vi "Refocus.vi"(8 "Error In":errorcluster, 11 "Focus and Tracking":T1) -> (0 "Error Out":errorcluster, 2 "Error":bool)   [LabVIEW 2012, in "Targeting Unit.lvlib"]
uses:
  Targeting Unit.lvlib
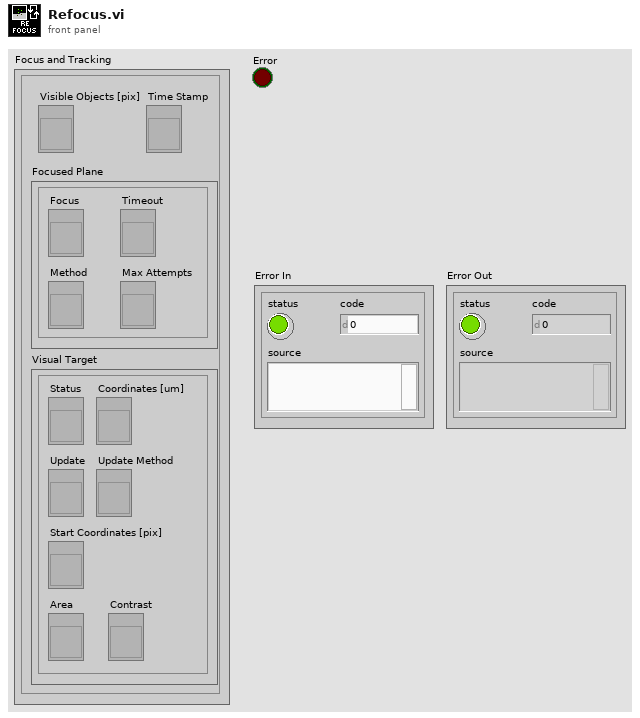
[diagram p1: front panel]
types:
  T1 = cluster{"Focused Plane":cluster{"Focus":refnum<vi>, "Timeout":refnum<vi>, "Max Attempts":refnum<vi>, "Method":refnum<vi>}, "Time Stamp":refnum<vi>, "Visual Target":cluster{"Coordinates [um]":refnum<vi>, "Status":refnum<vi>, "Update":refnum<vi>, "Update Method":refnum<vi>, "Start Coordinates [pix]":refnum<vi>, "Area":refnum<vi>, "Contrast":refnum<vi>}, "Visible Objects [pix]":refnum<vi>}
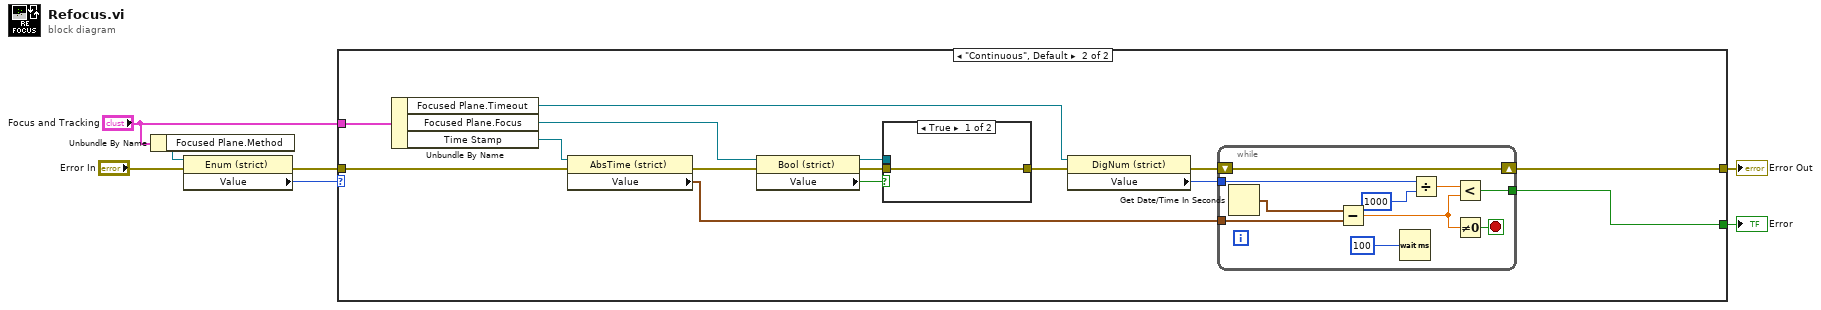
[diagram p0: block diagram]
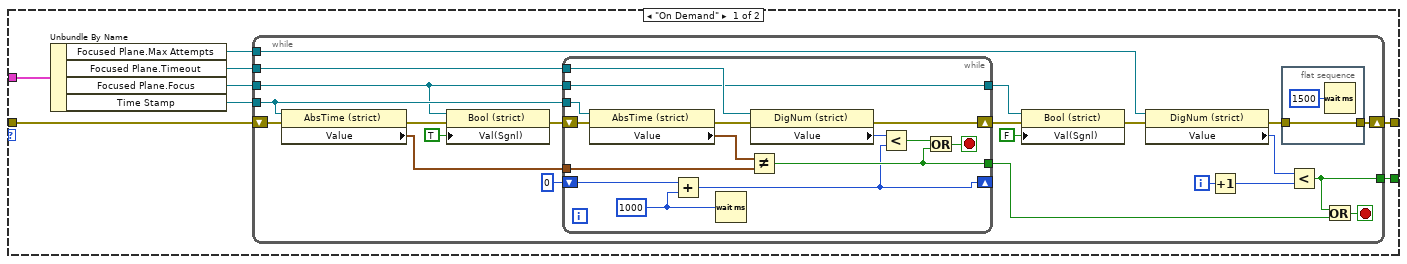
[diagram p2: hidden frame]
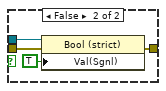
[diagram p3: hidden frame]
diagram:
  n1 = Unbundle By Name("Focus and Tracking") -> ("Focused Plane.Method"=w5:refnum<vi>)
  n2 = property class="Enum (strict)"(reference=w5, error in="Error In") -> (error out=w3:errorcluster, "Value"=w2:enum16{"Continuous", "On Demand"})  [unwired: 1 out]
  n3 = case shown="\"Continuous\", Default" w2 {
    tunnel: [w15 w69] -> w7
    tunnel: w3 -> [w14 w66]
    tunnel: [w13 w68] -> w6
    tunnel: "Focus and Tracking" -> [w12 w67]
    frame "On Demand" {
      n4 = Unbundle By Name(w12) -> ("Focused Plane.Max Attempts"=w8:refnum<vi>, "Focused Plane.Timeout"=w9:refnum<vi>, "Focused Plane.Focus"=w10:refnum<vi>, "Time Stamp"=w11:refnum<vi>)
      n5 = while {
        tunnel: w10 -> [w19]
        tunnel: w11 -> [w20]
        shift-right: [w17] -> w13
        shift-left: w14 -> [w23]
        tunnel: w8 -> [w29]
        tunnel: w9 -> [w27]
        tunnel: [w24] -> w15
        i -> [w32]
        stop <- w30 stop-if-true
        n6 = property class="AbsTime (strict)"(reference=w20, error in=w23) -> (error out=w22:errorcluster, "Value"=w21:timestamp)  [unwired: 1 out]
        n7 = property class="Bool (strict)"(reference=w19, error in=w22, "Val(Sgnl)"=TRUE ("Value (Signaling)")) -> (error out=w36:errorcluster)  [unwired: 1 out]
        n8 = while {
          tunnel: w21 -> [w53]
          tunnel: w20 -> [w52]
          shift-right: [w42] -> _
          shift-left: u32 0 -> [w43]
          tunnel: [w50] -> w18
          shift-right: [w48] -> w34
          shift-left: w36 -> [w54]
          tunnel: w27 -> [w47]
          tunnel: [w46] -> w26
          tunnel: w19 -> [w46]
          stop <- w51 stop-if-true
          w40 = u32 1000 ("milliseconds to wait")
          n9 = property class="AbsTime (strict)"(reference=w52, error in=w54) -> (error out=w49:errorcluster, "Value"=w41:timestamp)  [unwired: 1 out]
          n10 = Add(x=w43, y=w40) -> (x+y=w42:u32)
          n11 = Wait (ms)(milliseconds to wait=w40) -> ()  [unwired: 1 out]
          n12 = Not Equal?(x=w41, y=w53) -> (x != y?=w50:bool)
          n13 = property class="DigNum (strict)"(reference=w47, error in=w49) -> (error out=w48:errorcluster, "Value"=w45:u32)  [unwired: 1 out]
          n14 = Less?(x=w45, y=w42) -> (x < y?=w44:bool)
          n15 = Or(x=w44, y=w50) -> (x .or. y?=w51:bool)
        }
        n16 = property class="Bool (strict)"(reference=w26, error in=w34, "Val(Sgnl)"=FALSE ("Value (Signaling)")) -> (error out=w25:errorcluster)  [unwired: 1 out]
        n17 = property class="DigNum (strict)"(reference=w29, error in=w25) -> (error out=w16:errorcluster, "Value"=w28:u32)  [unwired: 1 out]
        n18 = Increment(x=w32) -> (x+1=w31:i32)
        n19 = flat-sequence {
          tunnel: [w38] -> w17
          tunnel: w16 -> [w38]
          frame #0 {
            n20 = Wait (ms)(milliseconds to wait=u32 1500) -> ()  [unwired: 1 out]
          }
        }
        n21 = Less?(x=w28, y=w31) -> (x < y?=w24:bool)
        n22 = Or(x=w24, y=w18) -> (x .or. y?=w30:bool)
      }
    }
    frame "Continuous", Default {
      n23 = Unbundle By Name(w67) -> ("Focused Plane.Timeout"=w56:refnum<vi>, "Focused Plane.Focus"=w60:refnum<vi>, "Time Stamp"=w65:refnum<vi>)
      n24 = property class="AbsTime (strict)"(reference=w65, error in=w66) -> (error out=w63:errorcluster, "Value"=w64:timestamp)  [unwired: 1 out]
      n25 = property class="Bool (strict)"(reference=w60, error in=w63) -> (reference out=w61:refnum<vi>, error out=w62:errorcluster, "Value"=w59:bool)
      n26 = case shown="True" w59 {
        tunnel: [w70 w74] -> w58
        tunnel: w62 -> [w70 w73]
        tunnel: w61 -> [_ w72]
        frame True {
        }
        frame False {
          n27 = property class="Bool (strict)"(reference=w72, error in=w73, "Val(Sgnl)"=TRUE ("Value (Signaling)")) -> (error out=w74:errorcluster)  [unwired: 1 out]
        }
      }
      n28 = property class="DigNum (strict)"(reference=w56, error in=w58) -> (error out=w57:errorcluster, "Value"=w55:u32)  [unwired: 1 out]
      n29 = while {
        shift-right: [w76] -> w68
        shift-left: w57 -> [w76]
        tunnel: [w84] -> w69
        tunnel: w64 -> [w78]
        tunnel: w55 -> [w75]
        stop <- w82 stop-if-true
        n30 = Get Date/Time In Seconds() -> (seconds since 1Jan1904=w77:timestamp)
        n31 = Subtract(x=w77, y=w78) -> (x-y=w83:dbl)
        n32 = Wait (ms)(milliseconds to wait=u32 100) -> ()  [unwired: 1 out]
        n33 = Divide(x=w75, y=u32 1000) -> (x/y=w81:dbl)
        n34 = Less?(x=w81, y=w83) -> (x < y?=w84:bool)
        n35 = Not Equal To 0?(x=w83) -> (x != 0?=w82:bool)
      }
    }
  }
  "Error" <- w7
  "Error Out" <- w6
